vi "PROXY_send_reference_updated_to_PLCs.vi"(8 "error_in":errorcluster, 11 "all_config_info_out":T1) -> (0 "error_out":errorcluster)   [LabVIEW 2020]
uses:
  ini/typedef/PROXY_all_config_info.ctl
  ini/typedef/PROXY_main_ini_file.ctl
  queues/typedef/PROXY_queue_refnums.ctl
  queues/typedef/STATION_queue_element.ctl
  STATION/ST_SQL_sequence_state.ctl
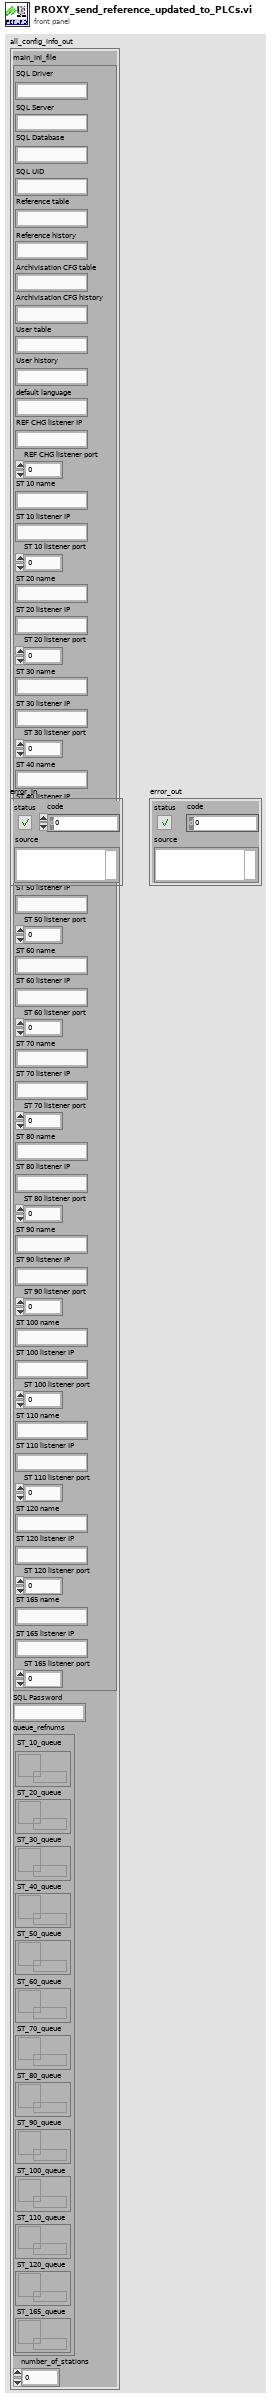
[diagram p1: front panel]
types:
  T1 = typedef "PROXY_all_config_info.ctl" = cluster{"main_ini_file":T2, "SQL Password":string, "queue_refnums":T3, "number_of_stations":i32}
  T2 = typedef "PROXY_main_ini_file.ctl" = cluster{"SQL Driver":string, "SQL Server":string, "SQL Database":string, "SQL UID":string, "Reference table":string, "Reference history":string, "Archivisation CFG table":string, "Archivisation CFG history":string, "User table":string, "User history":string, "default language":string, "REF CHG listener IP":string, "REF CHG listener port":u16, "ST 10 name":string, "ST 10 listener IP":string, "ST 10 listener port":u16, "ST 20 name":string, "ST 20 listener IP":string, "ST 20 listener port":u16, "ST 30 name":string, "ST 30 listener IP":string, "ST 30 listener port":u16, "ST 40 name":string, "ST 40 listener IP":string, "ST 40 listener port":u16, "ST 50 name":string, "ST 50 listener IP":string, "ST 50 listener port":u16, "ST 60 name":string, "ST 60 listener IP":string, "ST 60 listener port":u16, "ST 70 name":string, "ST 70 listener IP":string, "ST 70 listener port":u16, "ST 80 name":string, "ST 80 listener IP":string, "ST 80 listener port":u16, "ST 90 name":string, "ST 90 listener IP":string, "ST 90 listener port":u16, "ST 100 name":string, "ST 100 listener IP":string, "ST 100 listener port":u16, "ST 110 name":string, "ST 110 listener IP":string, "ST 110 listener port":u16, "ST 120 name":string, "ST 120 listener IP":string, "ST 120 listener port":u16, "ST 165 name":string, "ST 165 listener IP":string, "ST 165 listener port":u16}
  T3 = typedef "PROXY_queue_refnums.ctl" = cluster{"ST_10_queue":refnum<queue>, "ST_20_queue":refnum<queue>, "ST_30_queue":refnum<queue>, "ST_40_queue":refnum<queue>, "ST_50_queue":refnum<queue>, "ST_60_queue":refnum<queue>, "ST_70_queue":refnum<queue>, "ST_80_queue":refnum<queue>, "ST_90_queue":refnum<queue>, "ST_100_queue":refnum<queue>, "ST_110_queue":refnum<queue>, "ST_120_queue":refnum<queue>, "ST_165_queue":refnum<queue>}
  T4 = typedef "STATION_queue_element.ctl" = cluster{"state":T5, "variable":variant}
  T5 = typedef "ST_SQL_sequence_state.ctl" = enum16{"initialize", "get_next_state", "send_to_SQL", "send_to_PLC", "error", "stop"}
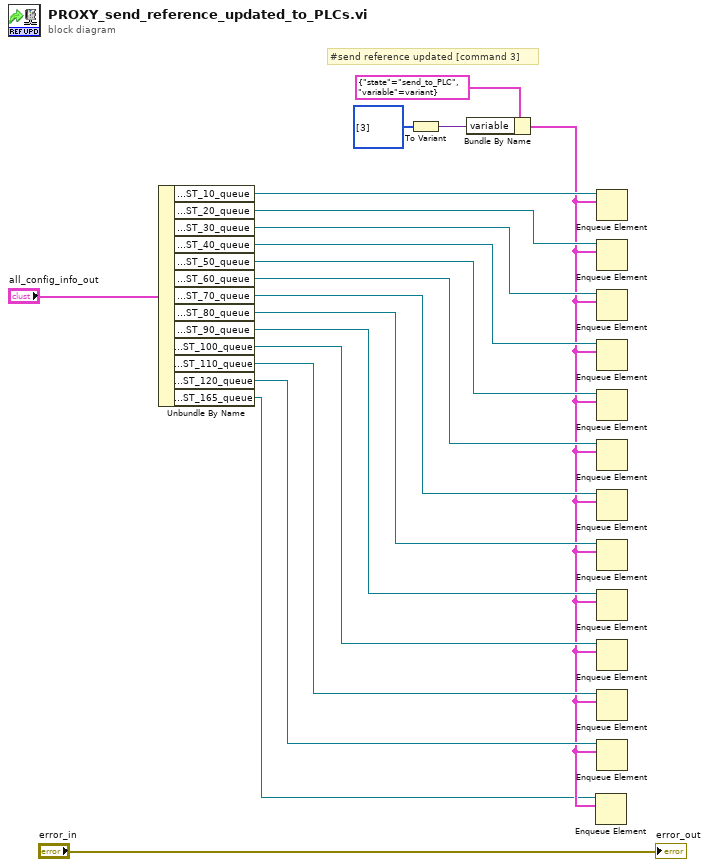
[diagram p0: block diagram]
diagram:
  # "#send reference updated [command 3]"
  n1 = Unbundle By Name("all_config_info_out") -> ("queue_refnums.ST_10_queue"=w18:refnum<queue>, "queue_refnums.ST_20_queue"=w14:refnum<queue>, "queue_refnums.ST_30_queue"=w13:refnum<queue>, "queue_refnums.ST_40_queue"=w11:refnum<queue>, "queue_refnums.ST_50_queue"=w10:refnum<queue>, "queue_refnums.ST_60_queue"=w9:refnum<queue>, "queue_refnums.ST_70_queue"=w6:refnum<queue>, "queue_refnums.ST_80_queue"=w8:refnum<queue>, "queue_refnums.ST_90_queue"=w7:refnum<queue>, "queue_refnums.ST_100_queue"=w5:refnum<queue>, "queue_refnums.ST_110_queue"=w4:refnum<queue>, "queue_refnums.ST_120_queue"=w3:refnum<queue>, "queue_refnums.ST_165_queue"=w1:refnum<queue>)
  n2 = To Variant(anything=u8[] [3]) -> (Variant=w15:variant)
  n3 = Bundle By Name(cluster=T4 {"state"=enum."send_to_PLC", "variable"=variant} ("element"), "variable"=w15) -> (w2:T4)
  n4 = Enqueue Element(queue=w1, element=w2) -> ()  [unwired: 2 in, 3 out]
  n5 = Enqueue Element(queue=w18, element=w2) -> ()  [unwired: 2 in, 3 out]
  n6 = Enqueue Element(queue=w14, element=w2) -> ()  [unwired: 2 in, 3 out]
  n7 = Enqueue Element(queue=w13, element=w2) -> ()  [unwired: 2 in, 3 out]
  n8 = Enqueue Element(queue=w11, element=w2) -> ()  [unwired: 2 in, 3 out]
  n9 = Enqueue Element(queue=w10, element=w2) -> ()  [unwired: 2 in, 3 out]
  n10 = Enqueue Element(queue=w9, element=w2) -> ()  [unwired: 2 in, 3 out]
  n11 = Enqueue Element(queue=w6, element=w2) -> ()  [unwired: 2 in, 3 out]
  n12 = Enqueue Element(queue=w8, element=w2) -> ()  [unwired: 2 in, 3 out]
  n13 = Enqueue Element(queue=w7, element=w2) -> ()  [unwired: 2 in, 3 out]
  n14 = Enqueue Element(queue=w5, element=w2) -> ()  [unwired: 2 in, 3 out]
  n15 = Enqueue Element(queue=w4, element=w2) -> ()  [unwired: 2 in, 3 out]
  n16 = Enqueue Element(queue=w3, element=w2) -> ()  [unwired: 2 in, 3 out]
  "error_out" <- "error_in"
